vi "Get Configuration Settings.vi"(8 "error in (no error)":errorcluster) -> (0 "error out":errorcluster, 3 "Acquisition and Logging Configuration":T1={"Thresholds"=[], "Epics Configuration"={"Input active"=[], "# Samples Post Trig"=4, "Armed"=FALSE}, "Epics Configuration File"="", "Number of Channels"=0.0, "Data rate"=0})   [LabVIEW 2014]
uses:
  controls/Master Configuration.ctl
  controls/EPICS Configuration.ctl
  <vilib>/Utility/xml.llb/Read From XML File(string).vi
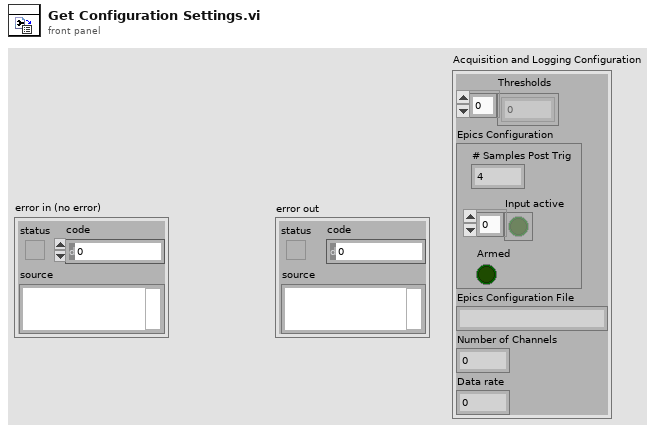
[diagram p1: front panel]
types:
  T1 = typedef "Master Configuration.ctl" = cluster{"Thresholds":dbl[], "Epics Configuration":T2, "Epics Configuration File":string, "Number of Channels":dbl, "Data rate":u32}
  T2 = typedef "EPICS Configuration.ctl" = cluster{"Input active":bool[], "# Samples Post Trig":u32, "Armed":bool}
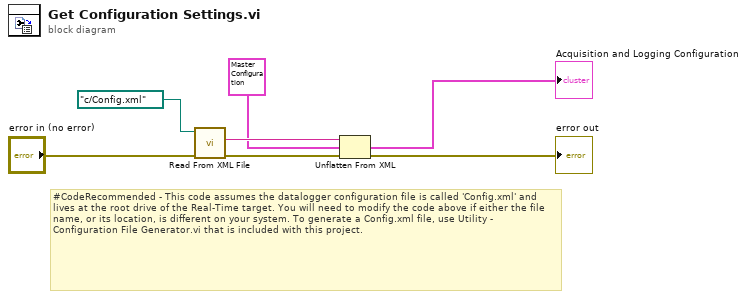
[diagram p0: block diagram]
diagram:
  # "#CodeRecommended - This code assumes the datalogger configuration file is called 'Config.xml' and lives at the root drive of the Real-Time target. You will need to modify the code above if either the file name, or its location, is different on your system. To generate a Config.xml file, use Utility - Configuration File Generator.vi that is included with this project."
  n1 = call-poly <vilib>:"Read From XML File.vi"("error in (no error)"="error in (no error)", "XML File Path"=path "c:/Config.xml") -> ("error out"=w6:errorcluster, "XML Elements"=w5:string)  [unwired: 7 in, 1 out]
  n2 = Unflatten From XML(xml string=w5, type=T1 {"Thresholds"=[], "Epics Configuration"={"Input active"=[], "# Samples Post Trig"=4, "Armed"=FALSE}, "Epics Configuration File"="c:\\EpicsConfig.cfg", "Number of Channels"=0.0, "Data rate"=0} ("Acquisition and Logging Configuration"), error in (no error)=w6) -> (value=→"Acquisition and Logging Configuration":T1, error out=→"error out":errorcluster)
